vi "Output Pin Initialization.vi"() -> (0 "error out":errorcluster, 1 "I/O Out Clock DAC (pin16)":refnum<k21>, 3 "I/O Out Clock ADC (pin17)":refnum<k21>)   [LabVIEW 2014]
doc: "This subVI enables the FPGA Digital output pin"
uses:
  <vilib>/rvi/eio/common/nirviEmuTemplateMethod_errors.vi
  <vilib>/eio/EIOMethodNode/EIOMethodNode.xnode
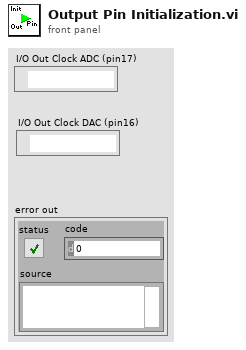
[diagram p1: front panel]
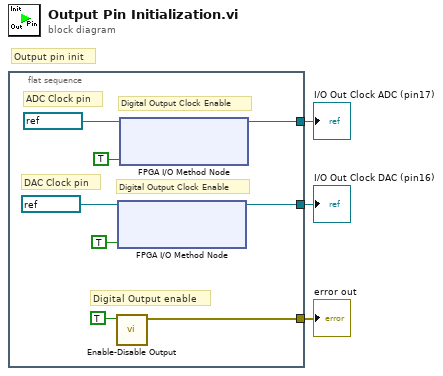
[diagram p0: block diagram]
diagram:
  # "Output pin init"
  n1 = flat-sequence {
    tunnel: [w9] -> w3
    tunnel: [w7] -> w1
    tunnel: [w4] -> w2
    frame #0 {
      # "Digital Output Clock Enable"
      # "DAC Clock pin"
      # "Digital Output Clock Enable"
      # "Digital Output enable"
      # "ADC Clock pin"
      n2 = call "Enable-Disable Output.vi"("Enable"=TRUE) -> ("error out"=w7:errorcluster)  [unwired: 10 in]
      n3 = xnode "FPGA I/O Method Node"("FPGA I/O In"=refnum<k21> "DIO16", "Enable"=TRUE) -> ("FPGA I/O Out"=w4:refnum<k21>)
      n4 = xnode "FPGA I/O Method Node"("FPGA I/O In"=refnum<k21> "DIO17", "Enable"=TRUE) -> ("FPGA I/O Out"=w9:refnum<k21>)
    }
  }
  "I/O Out Clock ADC (pin17)" <- w3
  "I/O Out Clock DAC (pin16)" <- w2
  "error out" <- w1
